vi "GetSpeedCmd (1).vi"(11 "Speed":dbl) -> (3 "Cmds":string[](array[string]))   [LabVIEW 2013]
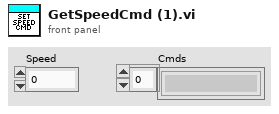
[diagram p1: front panel]
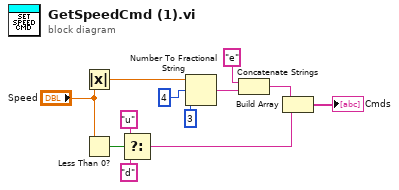
[diagram p0: block diagram]
diagram:
  n1 = Absolute Value(x="Speed") -> (abs(x)=w1:dbl)
  n2 = Less Than 0?(x="Speed") -> (x < 0?=w3:bool)
  n3 = Select(t="u", s=w3, f="d") -> (s? t:f=w11:string)
  n4 = Number To Fractional String(number=w1, width (-)=i16 4, precision (6)=i16 3 ("width (-)")) -> (F-format string=w9:string)  [unwired: 1 in]
  n5 = Concatenate Strings("e", w9) -> (w10:string)
  n6 = Build Array(w10, w11) -> (→"Cmds":string[])
